vi "DestroyPriorityQueue.vi"(8 "error in (no error)":errorcluster, 11 "Queue":refnum<data-value>) -> (0 "error out":errorcluster)   [LabVIEW 2009, in "PriorityQueue.lvlib"]
uses:
  PriorityQueue.lvlib
  PriorityQueue/PriorityQueue.lvclass
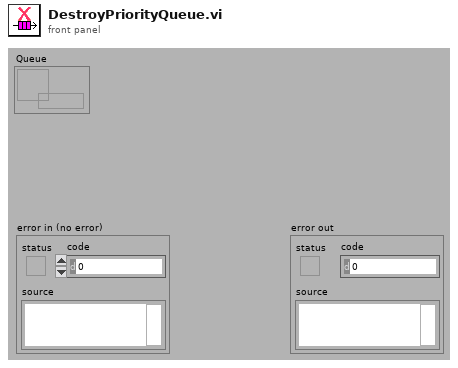
[diagram p1: front panel]
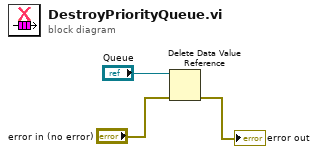
[diagram p0: block diagram]
diagram:
  n1 = Delete Data Value Reference(data value reference="Queue", error in="error in (no error)") -> (error out=→"error out":errorcluster)  [unwired: 1 out]
